vi "fix_path_os.vi"() -> ()   [LabVIEW 2013]
panel:
  out "name":string
  out "stripped path":path
  out "Path":path
  in  "path_string":string
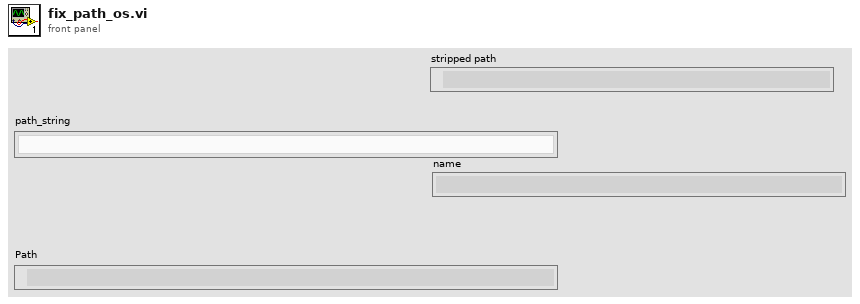
[diagram p1: front panel]
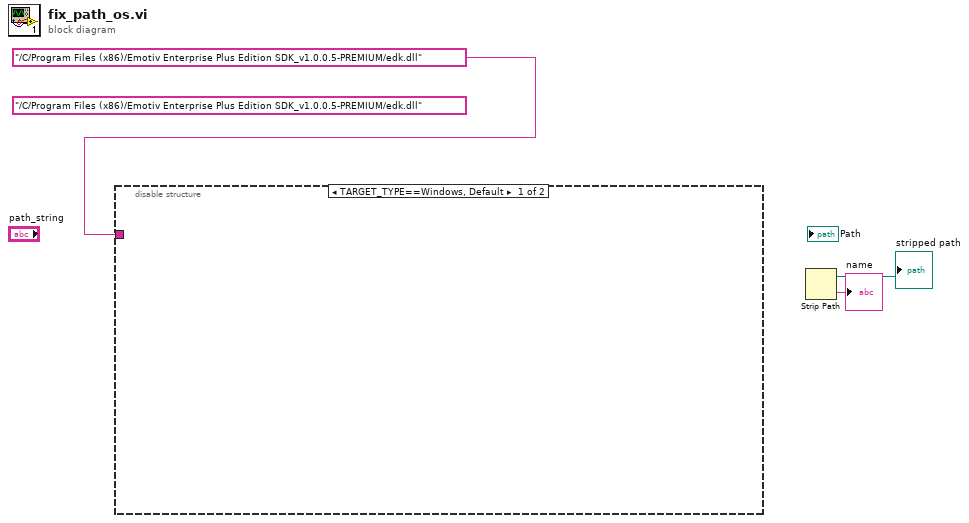
[diagram p0: block diagram]
diagram:
  (unwired) "/C/Program Files (x86)/Emotiv Enterprise Plus Edition SDK_v1.0.0.5-PREMIUM/edk.dll"
  n1 = disable-structure shown="TARGET_TYPE==Windows, Default" {
    disable-tunnel: "/C/Program Files (x86)/Emotiv Enterprise Plus Edition SDK_v1.0.0.5-PREMIUM/edk.dll" -> [_ _]
    frame condition #0 (active) {
    }
    frame condition #1 {
    }
  }
  n2 = Strip Path() -> (stripped path=→"stripped path":path, name=→"name":string)  [unwired: 1 in]
